vi "Speak withDPO-4034 (SUBVI)2.0.vi"(2 "Send Command":string, 3 "Send:  TRUE\nRecive: FALSE":bool, 4 "VISA Resource Name":refnum<visa-resource-name>) -> (0 "error out":errorcluster, 1 "Read Buffer":string)   [LabVIEW 2010]
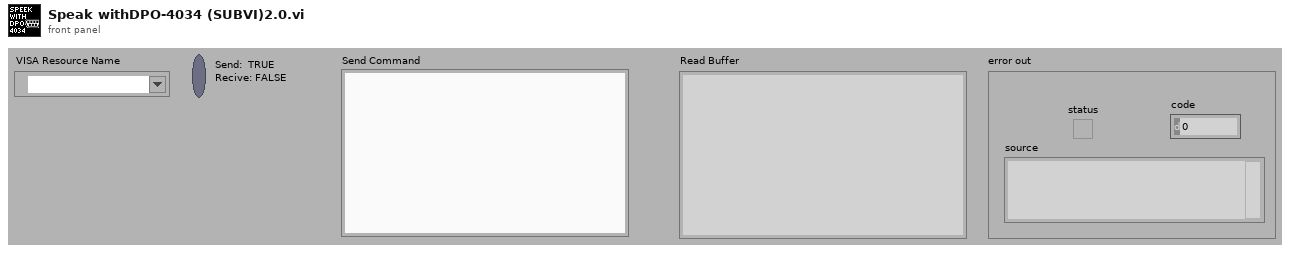
[diagram p1: front panel]
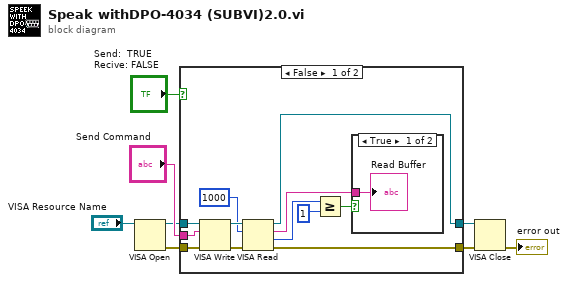
[diagram p0: block diagram]
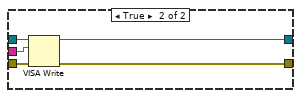
[diagram p3: hidden frame]
diagram:
  n1 = VISA Open(VISA resource name="VISA Resource Name") -> (VISA resource name=w5:refnum<visa-resource-name>, error out=w4:errorcluster)  [unwired: 4 in]
  n2 = case shown="False" "Send:  TRUE\nRecive: FALSE" {
    tunnel: w5 -> [w17 w26]
    tunnel: w4 -> [w16 w25]
    tunnel: "Send Command" -> [w15 w22]
    tunnel: [w14 w24] -> w3
    tunnel: [w13 w23] -> w2
    frame False {
      n3 = VISA Write(VISA resource name=w17, write buffer=w15, error in (no error)=w16) -> (VISA resource name out=w19:refnum<visa-resource-name>, error out=w20:errorcluster)  [unwired: 1 out]
      n4 = VISA Read(VISA resource name=w19, byte count=1000 ("Byte tor read"), error in (no error)=w20) -> (VISA resource name out=w13:refnum<visa-resource-name>, read buffer=w12:string, return count=w11:u32, error out=w14:errorcluster)
      n5 = Greater Or Equal?(x=w11, y=1) -> (x >= y?=w9:bool)
      n6 = case shown="True" w9 {
        tunnel: w12 -> [w21 _]
        frame True {
          "Read Buffer" <- w21
        }
        frame False {
        }
      }
    }
    frame True {
      n7 = VISA Write(VISA resource name=w26, write buffer=w22, error in (no error)=w25) -> (VISA resource name out=w23:refnum<visa-resource-name>, error out=w24:errorcluster)  [unwired: 1 out]
    }
  }
  n8 = VISA Close(VISA resource name=w2, error in (no error)=w3) -> (error out=→"error out":errorcluster)
